vi "C State.vi"(0 "State":string="Initial?", 1 "Front Leg PS":bool=TRUE, 4 "Back Leg Up":bool, 5 "Mid Leg PS":bool=TRUE, 6 "Back Leg PS":bool=TRUE, 7 "Mid Leg Up":bool, 10 "Front Leg Up":bool, 11 "Back Claws Cmd":bool=TRUE, 13 "Front Claw Cmd":bool=TRUE) -> (20 "newState":string, 21 "Front Leg Cmd":enum16{"Down Closed", "Down Opened", "Up"}(ring), 22 "Drive Motor Enabled":bool=TRUE, 23 "Mid Leg Cmd":enum16{"Down Closed", "Down Opened", "Up"}(ring), 25 "Engage Back Leg":bool, 26 "Skids":bool)   [LabVIEW 2012]
uses:
  <vilib>/Rock Robotics/WPI/DriverStation/DriverStationLCD/WPI_DriverStationLCDLCDLine.ctl
  Begin/Global Variables.vi
panel:
  out "Error Text":string
  out "Console Msg":string
  out "Short Time Elapsed":bool caption="Time has Elapsed"
  out "Long Time Elapsed":bool
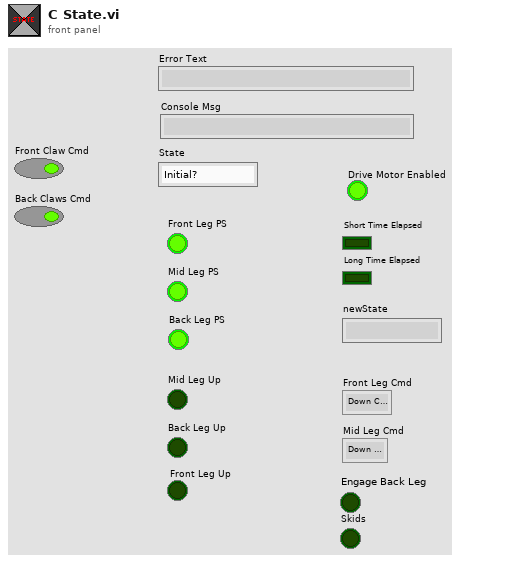
[diagram p1: front panel]
types:
  T1 = typedef "WPI_DriverStationLCDLCDLine.ctl" = enum16{"Main - Line 1", "User - Line 2", "User - Line 3", "User - Line 4", "User - Line 5", "User - Line 6"}
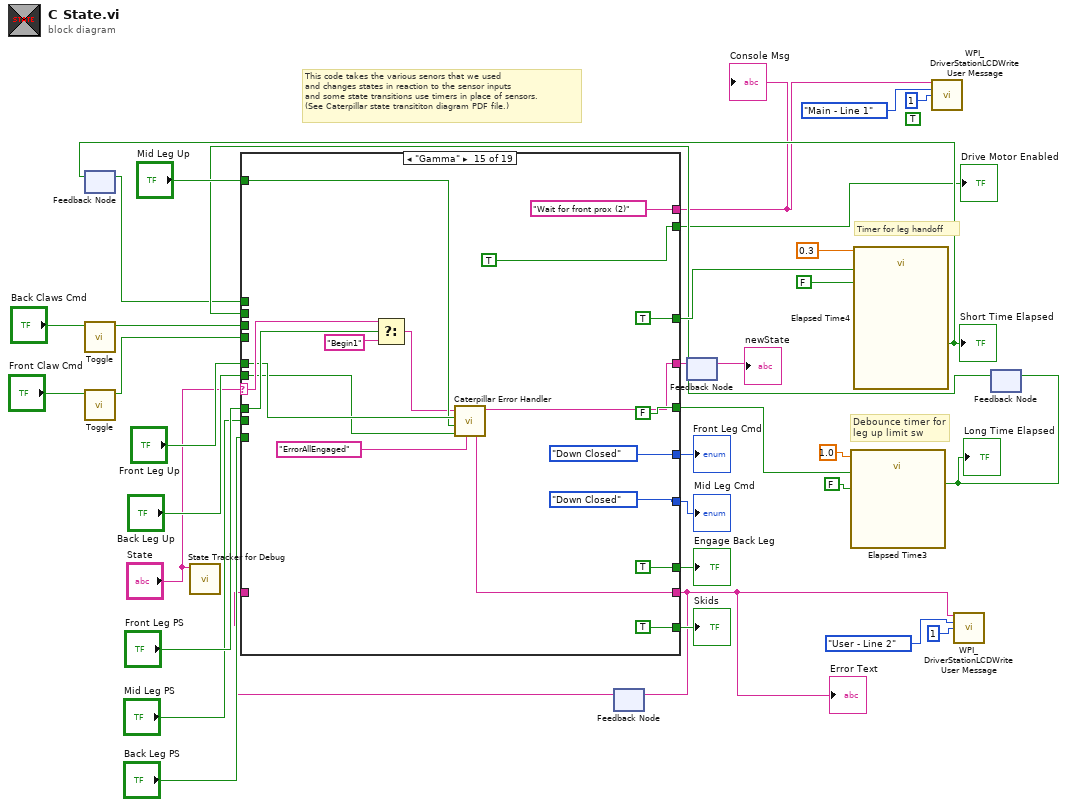
[diagram p0: block diagram]
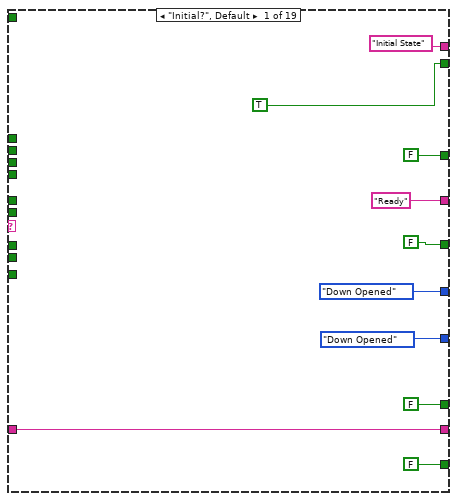
[diagram p2: hidden frame]
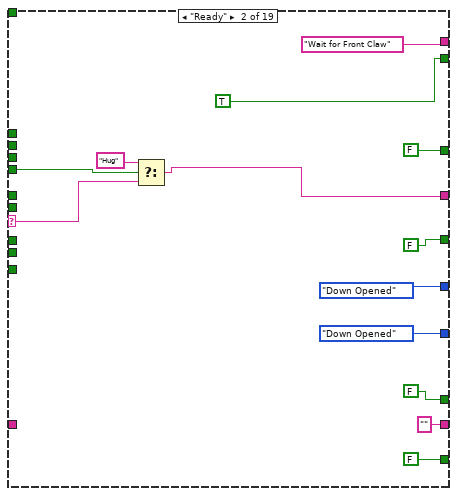
[diagram p3: hidden frame]
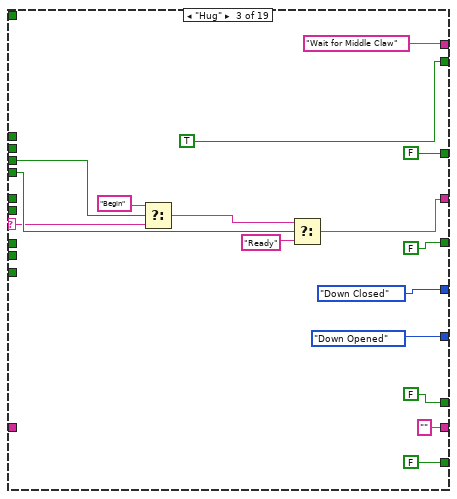
[diagram p4: hidden frame]
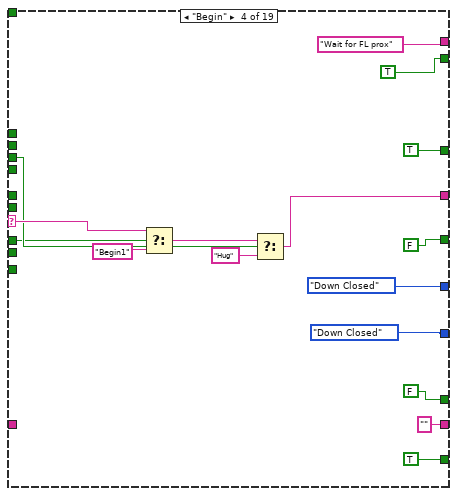
[diagram p5: hidden frame]
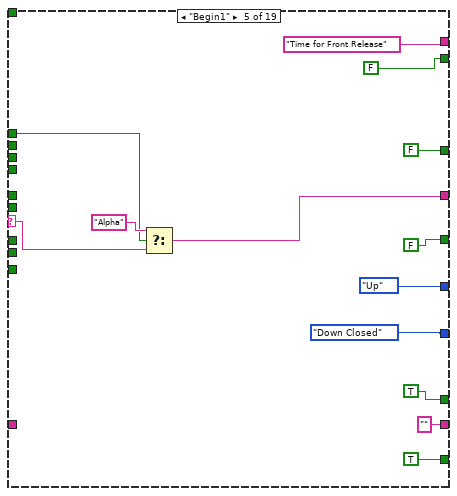
[diagram p6: hidden frame]
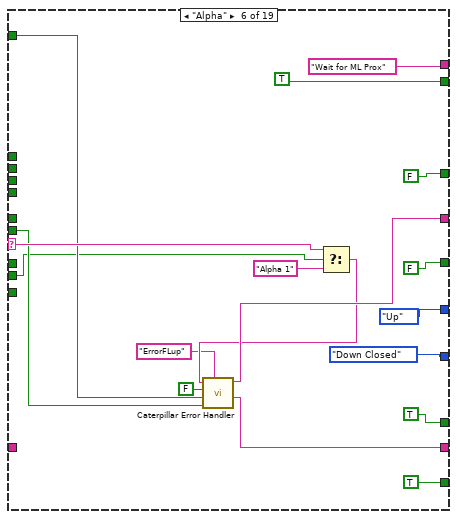
[diagram p7: hidden frame]
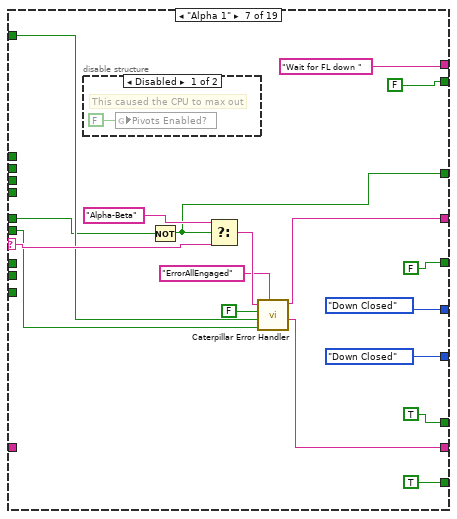
[diagram p8: hidden frame]
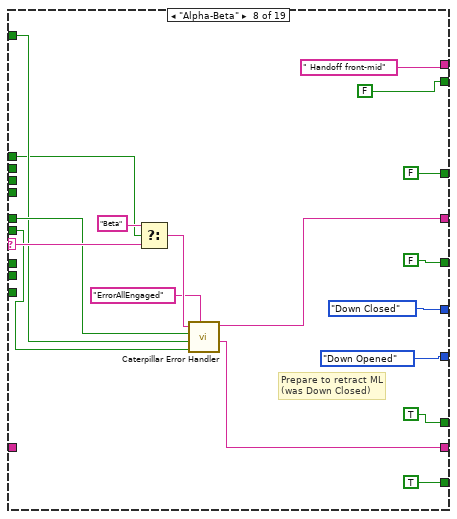
[diagram p10: hidden frame]
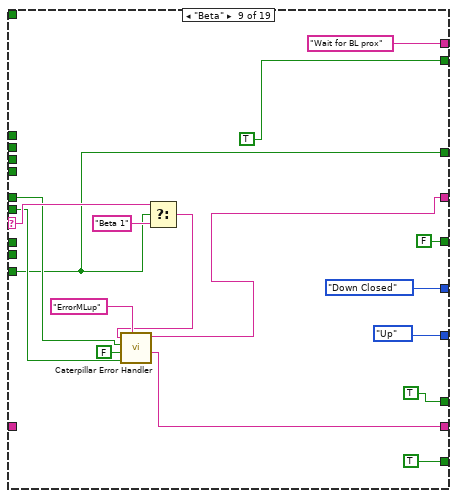
[diagram p11: hidden frame]
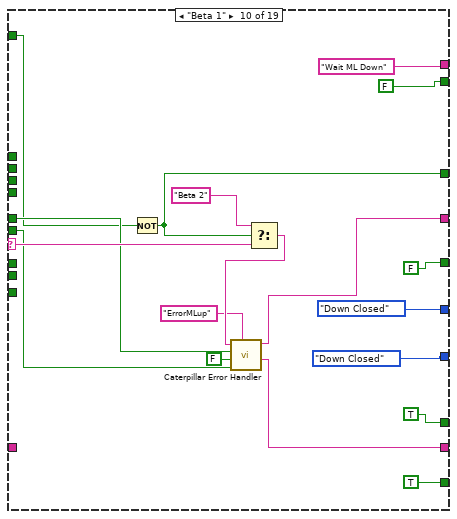
[diagram p12: hidden frame]
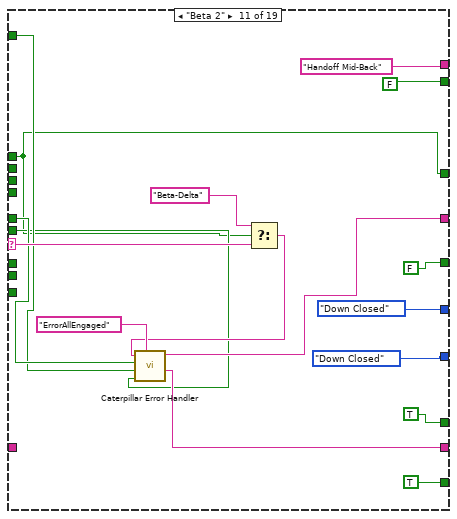
[diagram p13: hidden frame]
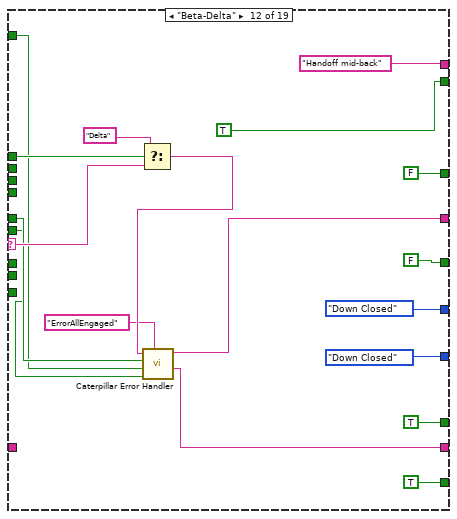
[diagram p14: hidden frame]
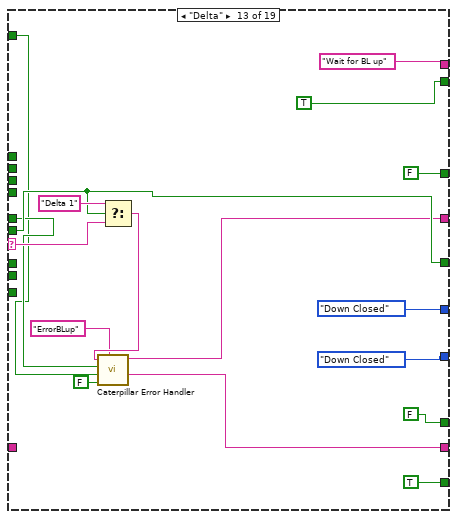
[diagram p15: hidden frame]
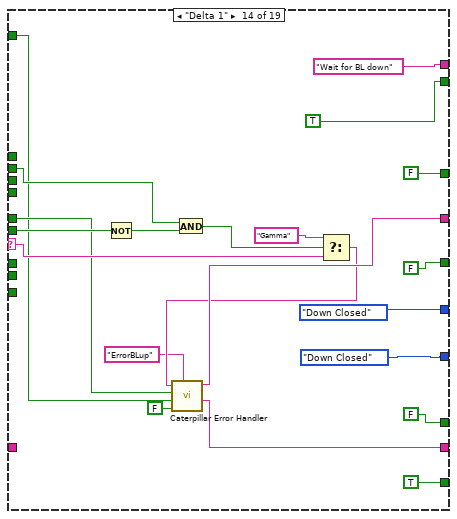
[diagram p16: hidden frame]
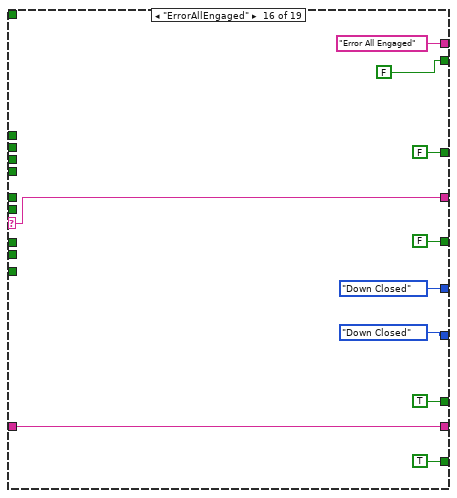
[diagram p17: hidden frame]
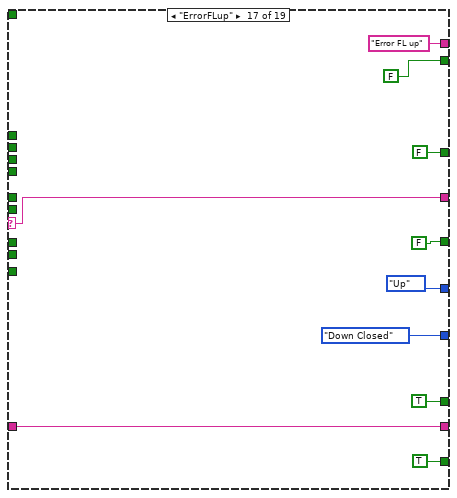
[diagram p18: hidden frame]
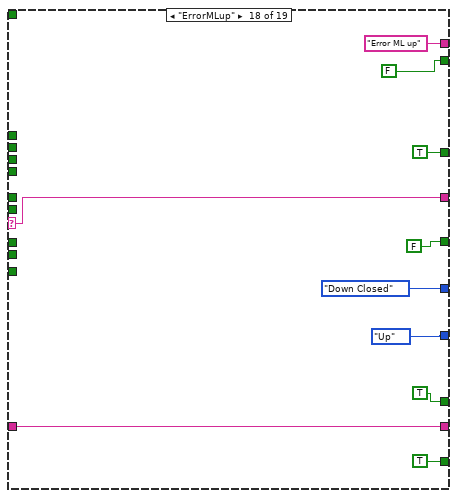
[diagram p19: hidden frame]
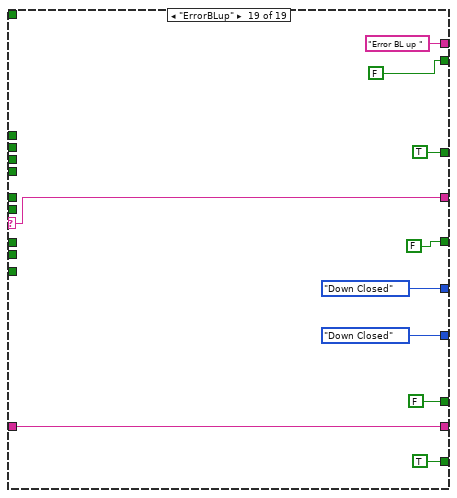
[diagram p20: hidden frame]
diagram:
  (unwired) TRUE ("clear line before write (T)")
  # "This code takes the various senors that we used\nand changes states in reaction to the sensor inputs\nand some state transitions use timers in place of sensors.\n(See Caterpillar state transititon diagram PDF file.)"
  # "Timer for leg handoff"
  # "Debounce timer for \nleg up limit sw"
  n1 = feedback #1() -> (w17:bool)  [unwired: 1 in]
  n2 = call "Toggle.vi"("Boolean"="Back Claws Cmd") -> ("Toggled"=w15:bool)  [unwired: 10 in]
  n3 = call "Toggle.vi"("Boolean"="Front Claw Cmd") -> ("Toggled"=w24:bool)  [unwired: 10 in]
  n4 = call "State Tracker for Debug.vi"("State"="State") -> ()  [unwired: 11 in]
  n5 = feedback #2() -> (w6:string)  [unwired: 1 in]
  n6 = feedback #3() -> (→"newState":string)  [unwired: 1 in]
  n7 = feedback #4() -> (w23:bool)  [unwired: 1 in]
  n8 = case shown="\"Gamma\"" "State" {
    selector: "State" -> [_ w56 w64 w84 w93 w119 w138 w156 w168 w190 w207 w225 w241 w257 w282 w291 w301 w311 w321]
    tunnel: ["Ready" ("t") w49 w61 w78 w94 w111 w130 w150 w165 w184 w200 w217 w235 w252 w274 w291 w301 w311 w321] -> w3
    tunnel: "Mid Leg PS" -> [_ _ _ _ _ w104 _ _ _ _ _ _ _ _ _ _ _ _ _]
    tunnel: "Front Leg PS" -> [_ _ _ w75 _ _ _ _ _ _ _ _ _ _ w281 _ _ _ _]
    tunnel: "Mid Leg Up" -> [_ _ _ _ _ w108 w129 w146 _ w179 w197 w213 w231 w248 w270 _ _ _ _]
    tunnel: "Back Leg Up" -> [_ _ _ _ _ w107 w128 w145 w161 w180 w196 w212 w240 w259 w271 _ _ _ _]
    tunnel: [FALSE FALSE ("clear line before write (T)") FALSE ("clear line before write (T)") FALSE ("clear line before write (T)") TRUE ("clear line before write (T)") TRUE ("clear line before write (T)") TRUE ("clear line before write (T)") TRUE ("clear line before write (T)") TRUE ("clear line before write (T)") TRUE ("clear line before write (T)") TRUE ("clear line before write (T)") TRUE ("clear line before write (T)") FALSE ("clear line before write (T)") FALSE ("clear line before write (T)") TRUE ("clear line before write (T)") TRUE ("clear line before write (T)") TRUE ("clear line before write (T)") TRUE ("clear line before write (T)") FALSE ("clear line before write (T)")] -> w33
    tunnel: [FALSE FALSE FALSE TRUE TRUE TRUE TRUE TRUE TRUE TRUE TRUE TRUE TRUE TRUE TRUE TRUE TRUE TRUE TRUE] -> w32
    tunnel: w17 -> [_ _ _ _ w91 _ _ w141 _ _ w194 w222 _ _ _ _ _ _ _]
    tunnel: [FALSE ("Time has Elapsed") FALSE ("Time has Elapsed") FALSE ("Time has Elapsed") TRUE ("Time has Elapsed") FALSE ("Time has Elapsed") FALSE ("Time has Elapsed") w123 FALSE ("Time has Elapsed") w159 w185 w194 FALSE ("Time has Elapsed") FALSE ("Time has Elapsed") FALSE ("Time has Elapsed") TRUE ("Time has Elapsed") FALSE ("Time has Elapsed") FALSE ("Time has Elapsed") TRUE ("Time has Elapsed") TRUE ("Time has Elapsed")] -> w28
    tunnel: w23 -> [_ _ _ _ _ _ _ _ _ _ _ _ _ w263 _ _ _ _ _]
    tunnel: [FALSE FALSE FALSE ("Back Leg Up") FALSE FALSE FALSE FALSE FALSE FALSE ("Back Leg Up") FALSE FALSE FALSE w240 FALSE FALSE FALSE ("Back Leg Up") FALSE ("Back Leg Up") FALSE ("Back Leg Up") FALSE ("Back Leg Up")] -> w21
    tunnel: "Front Leg Up" -> [_ _ _ _ _ _ w122 w147 w162 w181 w198 w214 w232 w249 w272 _ _ _ _]
    tunnel: [enum16{"Down Closed", "Down Opened", "Up"}."Down Opened" ("y") enum16{"Down Closed", "Down Opened", "Up"}."Down Opened" ("y") enum16{"Down Closed", "Down Opened", "Up"}."Down Closed" ("y") enum16{"Down Closed", "Down Opened", "Up"}."Down Closed" ("y") enum16{"Down Closed", "Down Opened", "Up"}."Up" ("y") enum16{"Down Closed", "Down Opened", "Up"}."Up" ("y") enum16{"Down Closed", "Down Opened", "Up"}."Down Closed" ("y") enum16{"Down Closed", "Down Opened", "Up"}."Down Closed" ("y") enum16{"Down Closed", "Down Opened", "Up"}."Down Closed" ("y") enum16{"Down Closed", "Down Opened", "Up"}."Down Closed" ("y") enum16{"Down Closed", "Down Opened", "Up"}."Down Closed" ("y") enum16{"Down Closed", "Down Opened", "Up"}."Down Closed" ("y") enum16{"Down Closed", "Down Opened", "Up"}."Down Closed" ("y") enum16{"Down Closed", "Down Opened", "Up"}."Down Closed" ("y") enum16{"Down Closed", "Down Opened", "Up"}."Down Closed" ("y") enum16{"Down Closed", "Down Opened", "Up"}."Down Closed" ("y") enum16{"Down Closed", "Down Opened", "Up"}."Up" ("y") enum16{"Down Closed", "Down Opened", "Up"}."Down Closed" ("y") enum16{"Down Closed", "Down Opened", "Up"}."Down Closed" ("y")] -> w26
    tunnel: w15 -> [_ _ w69 w83 _ _ _ _ _ _ _ _ _ _ _ _ _ _ _]
    tunnel: w24 -> [_ w46 w67 _ _ _ _ _ _ _ _ _ _ _ _ _ _ _ _]
    tunnel: "Back Leg PS" -> [_ _ _ _ _ _ _ _ w159 _ _ _ _ _ _ _ _ _ _]
    tunnel: [enum16{"Down Closed", "Down Opened", "Up"}."Down Opened" ("y") enum16{"Down Closed", "Down Opened", "Up"}."Down Opened" ("y") enum16{"Down Closed", "Down Opened", "Up"}."Down Opened" ("y") enum16{"Down Closed", "Down Opened", "Up"}."Down Closed" ("y") enum16{"Down Closed", "Down Opened", "Up"}."Down Closed" ("y") enum16{"Down Closed", "Down Opened", "Up"}."Down Closed" ("y") enum16{"Down Closed", "Down Opened", "Up"}."Down Closed" ("y") enum16{"Down Closed", "Down Opened", "Up"}."Down Opened" ("y") enum16{"Down Closed", "Down Opened", "Up"}."Up" ("Mid Leg Cmd") enum16{"Down Closed", "Down Opened", "Up"}."Down Closed" ("y") enum16{"Down Closed", "Down Opened", "Up"}."Down Closed" ("y") enum16{"Down Closed", "Down Opened", "Up"}."Down Closed" ("y") enum16{"Down Closed", "Down Opened", "Up"}."Down Closed" ("y") enum16{"Down Closed", "Down Opened", "Up"}."Down Closed" ("y") enum16{"Down Closed", "Down Opened", "Up"}."Down Closed" ("y") enum16{"Down Closed", "Down Opened", "Up"}."Down Closed" ("y") enum16{"Down Closed", "Down Opened", "Up"}."Down Closed" ("y") enum16{"Down Closed", "Down Opened", "Up"}."Up" ("y") enum16{"Down Closed", "Down Opened", "Up"}."Down Closed" ("y")] -> w13
    tunnel: ["Initial State" ("line text") "Wait for Front Claw" ("line text") "Wait for Middle Claw" ("line text") "Wait for FL prox" ("line text") "Time for Front Release" ("line text") "Wait for ML Prox" ("line text") "Wait for FL down " ("line text") " Handoff front-mid" ("line text") "Wait for BL prox" ("line text") "Wait ML Down" ("line text") "Handoff Mid-Back" ("line text") "Handoff mid-back" ("line text") "Wait for BL up" ("line text") "Wait for BL down" ("line text") "Wait for front prox (2)" ("line text") "Error All Engaged" ("line text") "Error FL up" ("line text") "Error ML up" ("line text") "Error BL up " ("line text")] -> w10
    tunnel: [w37 "" ("Error Text") "" ("Error Text") "" ("Error Text") "" ("Error Text") w112 w125 w143 w164 w178 w199 w216 w234 w253 w269 w286 w296 w306 w316] -> w5
    tunnel: w6 -> [w37 _ _ _ _ _ _ _ _ _ _ _ _ _ _ w286 w296 w306 w316]
    tunnel: [TRUE ("clear line before write (T)") TRUE ("clear line before write (T)") TRUE ("clear line before write (T)") TRUE ("clear line before write (T)") FALSE ("clear line before write (T)") TRUE ("clear line before write (T)") FALSE ("clear line before write (T)") FALSE ("clear line before write (T)") TRUE ("clear line before write (T)") FALSE ("clear line before write (T)") FALSE ("clear line before write (T)") TRUE ("clear line before write (T)") TRUE ("clear line before write (T)") TRUE ("clear line before write (T)") TRUE ("clear line before write (T)") FALSE ("clear line before write (T)") FALSE ("clear line before write (T)") FALSE ("clear line before write (T)") FALSE ("clear line before write (T)")] -> w4
    frame "Initial?", Default {
    }
    frame "Ready" {
      n9 = Select(t="Hug", s=w46, f=w56) -> (s? t:f=w49:string)
    }
    frame "Hug" {
      n10 = Select(t="Begin", s=w69, f=w64) -> (s? t:f=w65:string)
      n11 = Select(t=w65, s=w67, f="Ready" ("t")) -> (s? t:f=w61:string)
    }
    frame "Begin" {
      n12 = Select(t=w84, s=w75, f="Begin1") -> (s? t:f=w82:string)
      n13 = Select(t=w82, s=w83, f="Hug") -> (s? t:f=w78:string)
    }
    frame "Begin1" {
      n14 = Select(t="Alpha" ("f"), s=w91, f=w93) -> (s? t:f=w94:string)
    }
    frame "Alpha" {
      n15 = Select(t=w119, s=w104, f="Alpha 1") -> (s? t:f=w110:string)
      n16 = call "Caterpillar Error Handler.vi"("Error State"="ErrorFLup", "Back Leg Up"=w107, "Mid Leg Up"=w108, "Front Leg Up"=FALSE, "state in"=w110) -> ("Error Text"=w112:string, "state out"=w111:string)  [unwired: 5 in]
    }
    frame "Alpha 1" {
      n17 = disable-structure shown="Disabled" {
        frame Disabled {
          # "This caused the CPU to max out"
          n18 = global write "Global Variables.vi" "Pivots Enabled?"(FALSE ("Pivots Enabled?")) -> ()
        }
        frame Enabled {
        }
      }
      n19 = Not(x=w122) -> (.not. x?=w123:bool)
      n20 = Select(t="Alpha-Beta" ("f"), s=w123, f=w138) -> (s? t:f=w131:string)
      n21 = call "Caterpillar Error Handler.vi"("Error State"="ErrorAllEngaged", "Back Leg Up"=w128, "Mid Leg Up"=w129, "Front Leg Up"=FALSE, "state in"=w131) -> ("Error Text"=w125:string, "state out"=w130:string)  [unwired: 5 in]
    }
    frame "Alpha-Beta" {
      # "Prepare to retract ML\n(was Down Closed)"
      n22 = Select(t="Beta" ("f"), s=w141, f=w156) -> (s? t:f=w151:string)
      n23 = call "Caterpillar Error Handler.vi"("Error State"="ErrorAllEngaged", "Back Leg Up"=w145, "Mid Leg Up"=w146, "Front Leg Up"=w147, "state in"=w151) -> ("Error Text"=w143:string, "state out"=w150:string)  [unwired: 5 in]
    }
    frame "Beta" {
      n24 = Select(t=w168, s=w159, f="Beta 1") -> (s? t:f=w166:string)
      n25 = call "Caterpillar Error Handler.vi"("Error State"="ErrorMLup", "Back Leg Up"=w161, "Mid Leg Up"=FALSE, "Front Leg Up"=w162, "state in"=w166) -> ("Error Text"=w164:string, "state out"=w165:string)  [unwired: 5 in]
    }
    frame "Beta 1" {
      n26 = Not(x=w179) -> (.not. x?=w185:bool)
      n27 = Select(t="Beta 2" ("f"), s=w185, f=w190) -> (s? t:f=w183:string)
      n28 = call "Caterpillar Error Handler.vi"("Error State"="ErrorMLup", "Back Leg Up"=w180, "Mid Leg Up"=FALSE, "Front Leg Up"=w181, "state in"=w183) -> ("Error Text"=w178:string, "state out"=w184:string)  [unwired: 5 in]
    }
    frame "Beta 2" {
      n29 = Select(t="Beta-Delta" ("f"), s=w194, f=w207) -> (s? t:f=w201:string)
      n30 = call "Caterpillar Error Handler.vi"("Error State"="ErrorAllEngaged", "Back Leg Up"=w196, "Mid Leg Up"=w197, "Front Leg Up"=w198, "state in"=w201) -> ("Error Text"=w199:string, "state out"=w200:string)  [unwired: 5 in]
    }
    frame "Beta-Delta" {
      n31 = Select(t="Delta" ("f"), s=w222, f=w225) -> (s? t:f=w218:string)
      n32 = call "Caterpillar Error Handler.vi"("Error State"="ErrorAllEngaged", "Back Leg Up"=w212, "Mid Leg Up"=w213, "Front Leg Up"=w214, "state in"=w218) -> ("Error Text"=w216:string, "state out"=w217:string)  [unwired: 5 in]
    }
    frame "Delta" {
      n33 = Select(t="Delta 1" ("f"), s=w240, f=w241) -> (s? t:f=w236:string)
      n34 = call "Caterpillar Error Handler.vi"("Error State"="ErrorBLup", "Back Leg Up"=FALSE, "Mid Leg Up"=w231, "Front Leg Up"=w232, "state in"=w236) -> ("Error Text"=w234:string, "state out"=w235:string)  [unwired: 5 in]
    }
    frame "Delta 1" {
      n35 = Not(x=w259) -> (.not. x?=w260:bool)
      n36 = And(x=w263, y=w260) -> (x .and. y?=w262:bool)
      n37 = Select(t="Gamma" ("f"), s=w262, f=w257) -> (s? t:f=w251:string)
      n38 = call "Caterpillar Error Handler.vi"("Error State"="ErrorBLup", "Back Leg Up"=FALSE, "Mid Leg Up"=w248, "Front Leg Up"=w249, "state in"=w251) -> ("Error Text"=w253:string, "state out"=w252:string)  [unwired: 5 in]
    }
    frame "Gamma" {
      n39 = Select(t=w282, s=w281, f="Begin1") -> (s? t:f=w267:string)
      n40 = call "Caterpillar Error Handler.vi"("Error State"="ErrorAllEngaged", "Back Leg Up"=w271, "Mid Leg Up"=w270, "Front Leg Up"=w272, "state in"=w267) -> ("Error Text"=w269:string, "state out"=w274:string)  [unwired: 5 in]
    }
    frame "ErrorAllEngaged" {
    }
    frame "ErrorFLup" {
    }
    frame "ErrorMLup" {
    }
    frame "ErrorBLup" {
    }
  }
  "Engage Back Leg" <- w33
  "Skids" <- w32
  "Front Leg Cmd" <- w26
  "Mid Leg Cmd" <- w13
  "Console Msg" <- w10
  "Error Text" <- w5
  "Drive Motor Enabled" <- w4
  n41 = feedback-in #2(w5) -> ()
  n42 = feedback-in #3(w3) -> ()
  n43 = call "Elapsed Time3"("Time Target (s)"=1.0, "Reset"=w21, "Auto Reset"=FALSE) -> ("Time has Elapsed"=w22:bool)  [unwired: 9 in, 7 out]
  "Long Time Elapsed" <- w22
  n44 = call "Elapsed Time4"("Time Target (s)"=0.3, "Reset"=w28, "Auto Reset"=FALSE) -> ("Time has Elapsed"=w18:bool)  [unwired: 9 in, 7 out]
  "Short Time Elapsed" <- w18
  n45 = feedback-in #1(w18) -> ()
  n46 = call <vilib>:"WPI_DriverStationLCDWrite User Message.vi"("line text"=w10, "line"=WPI_DriverStationLCDLCDLine."Main - Line 1", "starting column"=i8 1) -> ()  [unwired: 12 in, 1 out]
  n47 = call <vilib>:"WPI_DriverStationLCDWrite User Message.vi"("line text"=w5, "line"=WPI_DriverStationLCDLCDLine."User - Line 2", "starting column"=i8 1) -> ()  [unwired: 12 in, 1 out]
  n48 = feedback-in #4(w22) -> ()
